vi "Fetch Digital Waveform Single.vi"(8 "error in (no error)":errorcluster {"code" format="%.0x"}, 10 "Channel Name (\"POD1\")":string(combo)="POD1", 11 "VISA Resource Name":refnum<visa-resource-name>) -> (0 "error out":errorcluster {"code" format="%.0x"}, 1 "x increment":dbl caption="x Increment" format="%^.2e", 2 "initial x":dbl caption="Initial x" format="%^.2e", 3 "VISA Resource Name Out":refnum<visa-resource-name>, 4 "waveform array":u16[](array[numeric]) caption="Waveform Array", 5 "actual points":u32 caption="Actual Points")   [LabVIEW 2011, in "Agilent 546XX Series.lvlib"]
doc: "This VI returns the waveform the oscilloscope acquires for the digital channel you specify. The waveform is from an acquisition that you previously initiated. \n\nYou use the ag546xx Initiate Acquisition VI to start an acquisition on the digital channels that you enable with the ag546xx Configure Digital Channel VI. The oscilloscope acquires waveforms for the enabled digital channels concurrently. You must call this VI separately for each enabled digital channel to obtain the waveforms.\n\nYou can call the ag546xx Read Digital Waveform VI instead of the ag546xx Initiate Acquisition VI. The ag546xx Read Digital Waveform VI starts an acquisition on all enabled channels, waits for the acquisition to complete, and returns the waveform for the channel you specify. You call this VI to obtain the digital waveforms for each of the remaining channels.\n\nNotes:\n\n(1) This VI returns the waveforms in PODs of digital channels 0 to 7 or 8 to 15.\n\n(2) The Waveform Array is returned as an unsigned 8 bit number with digital channels 7 or 15 as the most significant bit and digital channels 0 or 8 as the least significant bit, respectively. \n\n(3) This VI is only used by models 546xx\"D\" models."
uses:
  Agilent 546XX Series.lvlib
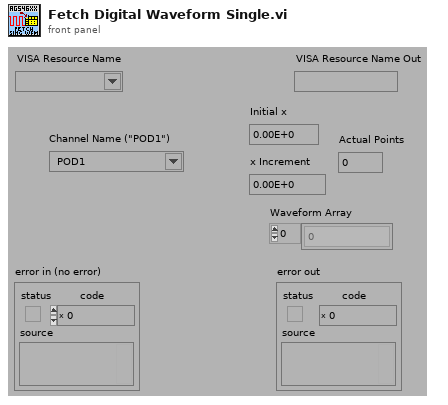
[diagram p1: front panel]
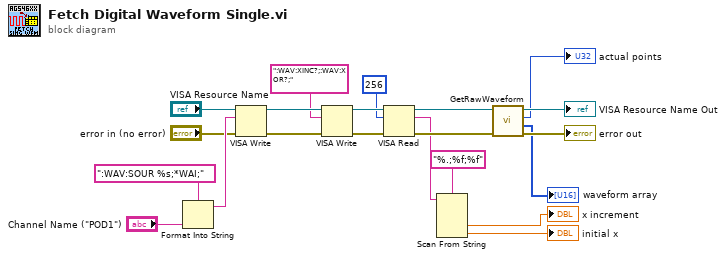
[diagram p0: block diagram]
diagram:
  n1 = Format Into String(format string=":WAV:SOUR %s;*WAI;", "Channel Name (\"POD1\")") -> (resulting string=w20:string)  [unwired: 2 in, 1 out]
  n2 = VISA Write(VISA resource name="VISA Resource Name", write buffer=w20, error in (no error)="error in (no error)") -> (VISA resource name out=w19:refnum<visa-resource-name>, error out=w18:errorcluster)  [unwired: 1 out]
  n3 = VISA Write(VISA resource name=w19, write buffer=":WAV:XINC?;:WAV:XOR?;", error in (no error)=w18) -> (VISA resource name out=w17:refnum<visa-resource-name>, error out=w16:errorcluster)  [unwired: 1 out]
  n4 = VISA Read(VISA resource name=w17, byte count=u32 256, error in (no error)=w16) -> (VISA resource name out=w15:refnum<visa-resource-name>, read buffer=w9:string, error out=w14:errorcluster)  [unwired: 1 out]
  n5 = Scan From String(format string="%.;%f;%f", input string=w9) -> (output 1=→"x increment":dbl, output 2=→"initial x":dbl)  [unwired: 4 in, 3 out]
  n6 = call "GetRawWaveform.vi"("error in"=w14, "VISA Resource Name"=w15) -> ("error out"=→"error out":errorcluster, "Waveform Array"=→"waveform array":u32[], "Number of Points"=→"actual points":u32, "VISA Resource Name Out"=→"VISA Resource Name Out":refnum<visa-resource-name>)  [unwired: 5 in, 1 out]
